vi "Feedback Node Demo.vi"() -> ()   [LabVIEW 2009]
uses:
  Instance           1 26Saved   Feedback Node Demo .vi
panel:
  out "shift register":dbl
  out "feedback Before":dbl
  out "feedback After":dbl
  in  "stop":bool
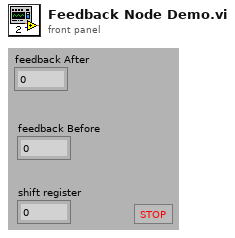
[diagram p1: front panel]
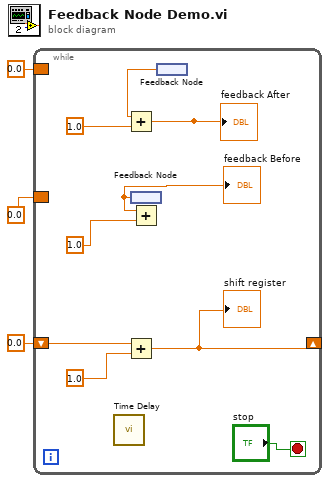
[diagram p0: block diagram]
diagram:
  n1 = while {
    shift-right: [w4] -> _
    shift-left: 0.0 -> [w5]
    border: 0.0 -> [_]
    border: 0.0 -> [_]
    stop <- "stop" stop-if-true
    n2 = call "Time Delay"() -> ()  [unwired: 11 in, 1 out]
    n3 = Add(x=w5, y=1.0) -> (x+y=w4:dbl)
    "shift register" <- w4
    n4 = feedback #1() -> (w7:dbl)
    "feedback Before" <- w7
    n5 = Add(x=w7, y=1.0) -> (x+y=w8:dbl)
    n6 = feedback #2() -> (w10:dbl)
    n7 = Add(x=w10, y=1.0) -> (x+y=w11:dbl)
    "feedback After" <- w11
  }
